vi "Query Control On.vi"(8 "error in (no error)":errorcluster, 11 "VISA resource name":refnum<visa-resource-name>="COM3") -> (0 "error out":errorcluster, 2 "Control on?":bool, 3 "VISA resource name out":refnum<visa-resource-name>)   [LabVIEW 2023]
panel:
  out "Current heater output":dbl
  out "Old set temperature":dbl
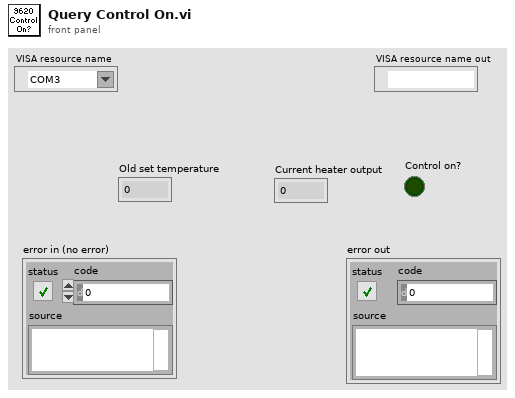
[diagram p1: front panel]
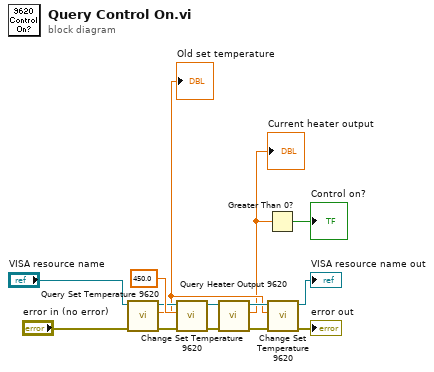
[diagram p0: block diagram]
diagram:
  n1 = call "Query Set Temperature 9620.vi"("error in (no error)"="error in (no error)", "VISA resource name"="VISA resource name") -> ("error out"=w11:errorcluster, "Set temperature"=w7:dbl, "VISA resource name out"=w10:refnum<visa-resource-name>)  [unwired: 7 in]
  "Old set temperature" <- w7
  n2 = call "Change Set Temperature 9620.vi"("error in (no error)"=w11, "Temperture Setpoint"=450.0, "VISA resource name"=w10) -> ("error out"=w1:errorcluster, "VISA resource name out"=w2:refnum<visa-resource-name>)  [unwired: 7 in]
  n3 = call "Query Heater Output 9620.vi"("error in (no error)"=w1, "VISA resource name"=w2) -> ("error out"=w8:errorcluster, "Current heater output"=w4:dbl, "VISA resource name out"=w9:refnum<visa-resource-name>)  [unwired: 7 in]
  "Current heater output" <- w4
  n4 = Greater Than 0?(x=w4) -> (x > 0?=→"Control on?":bool)
  n5 = call "Change Set Temperature 9620.vi"("error in (no error)"=w8, "Temperture Setpoint"=w7, "VISA resource name"=w9) -> ("error out"=→"error out":errorcluster, "VISA resource name out"=→"VISA resource name out":refnum<visa-resource-name>)  [unwired: 7 in]
